vi "Test Queue Log Provider.vi"() -> (1 "pass?":bool)   [LabVIEW 2019, in "ANODE Tests.lvlib"]
uses:
  ANODE Tests.lvlib
  ANODE/Utility API/Queue Log Provider/impl/log_message.ctl
  ANODE/Utility API/Log Service/public/level.ctl
  34bea0a4-f80a-4efe-aaf4-9db1f3a8a041.vi
  4e885d52-342e-4d6f-86c2-bbc79adb3db9.vi
  901ffbec-7f76-4fda-a8b3-ab898965128c.vi
  31a8342b-9139-4bdf-bbc1-bb92f7179d80.vi
  c69379c1-06bc-43e8-abf1-6b6e803fbc34.vi
  7ff86ca6-88c0-4de2-a7d7-e18e6c48d840.vi
  f5e9308b-311a-4c07-9062-c62029aec88d.vi
  cd498dcc-2004-4e95-9cb1-3a88910e2f61.vi
  4bbd3971-874f-4069-8a4a-00f2533dc096.vi
  51edfdbb-9a3d-492a-8a02-2d0f54c6b824.vi
  8f198e5f-b4d0-4ca0-822a-d58fe651c8a2.vi
  ANODE/Util/Timestamp or now.vi
  ANODE/Utility API/Queue Log Provider/Queue Log Provider.lvclass
  ANODE/Utility API/Log Service/Log Service.lvclass
panel:
  out "expected output?":bool
  out "expected # of elements?":bool
  out "remaining elements":T1[](array[typedef]) {"level" items=["OFF"=0, "FATAL"=100, "ERROR"=200, "WARN"=300, "INFO"=400, "DEBUG"=500, "TRACE"=600, "ALL"=65535]}
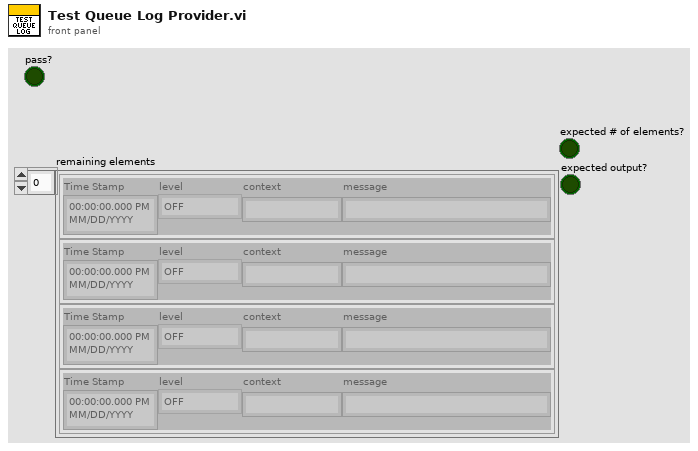
[diagram p1: front panel]
types:
  T1 = typedef "Utility API.lvlib/Queue Log Provider.lvclass/log_message.ctl" = cluster{"Time Stamp":timestamp, "level":T2, "context":string, "message":string}
  T2 = typedef "Utility API.lvlib/Log Service.lvclass/level.ctl" = u16
  T3 = typedef "LVCOOOP.lvlib/Support API.lvlib/Queue Log Provider.lvclass/log_message.ctl" = cluster{"Time Stamp":timestamp, "level":T4, "context":string, "message":string}
  T4 = typedef "LVCOOOP.lvlib/Support API.lvlib/Log Service.lvclass/level.ctl" = u16
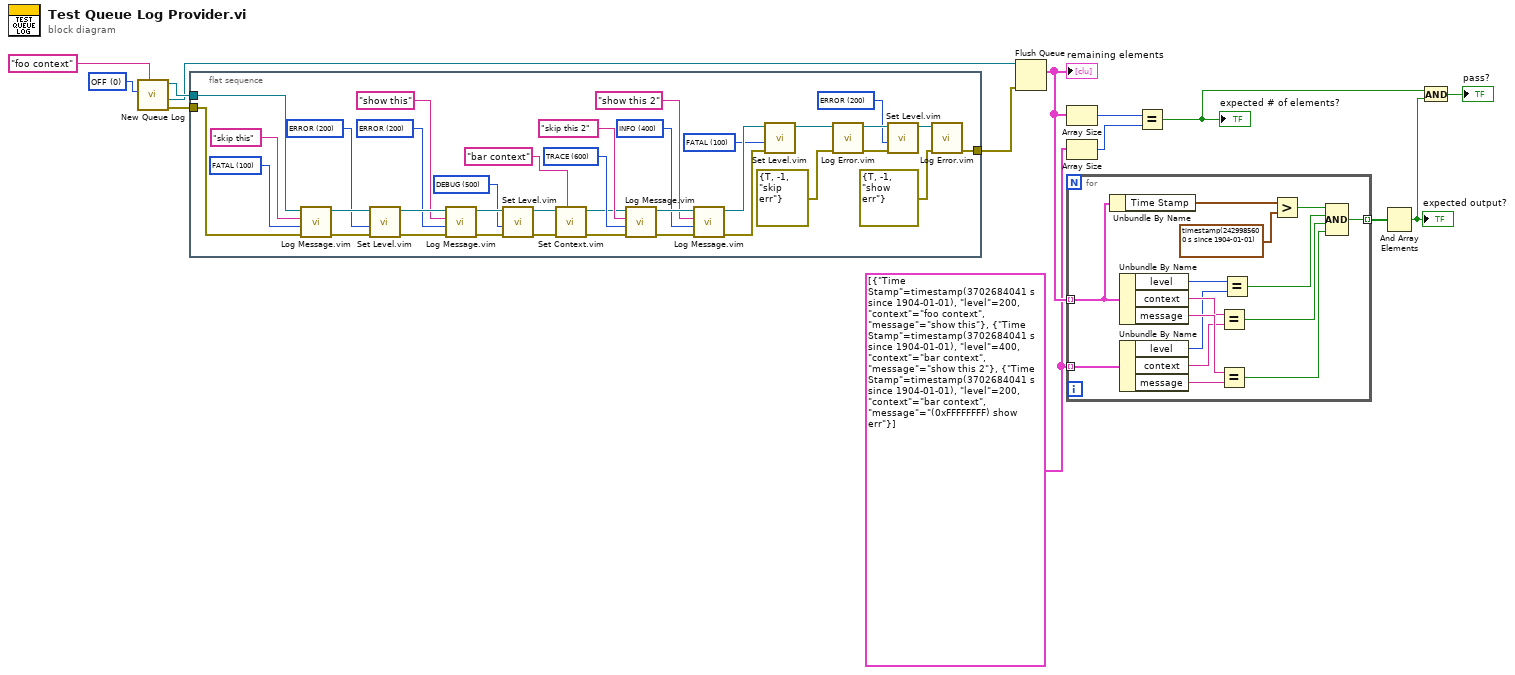
[diagram p0: block diagram]
diagram:
  w5 = T1[] [{"Time Stamp"=timestamp(3702684041.4619007 s since 1904-01-01), "level"=200, "context"="foo context", "message"="show this"}, {"Time Stamp"=timestamp(3702684041.4619007 s since 1904-01-01), "level"=400, "context"="bar context", "message"="show this 2"}, {"Time Stamp"=timestamp(3702684041.4619007 s since 1904-01-01), "level"=200, "context"="bar context", "message"="(0xFFFFFFFF) show err"}] ("remaining elements")
  w13 = T2 0 items=["OFF"=0, "FATAL"=100, "ERROR"=200, "WARN"=300, "INFO"=400, "DEBUG"=500, "TRACE"=600, "ALL"=65535] ("level")
  n1 = call "New Queue Log.vi"("context"="foo context", "level"=w13) -> ("error out"=w11:errorcluster, "queue out"=w9:refnum<queue>, "Queue Log Provider"=w12:refnum<data-value>)  [unwired: 7 in]
  n2 = flat-sequence {
    tunnel: w12 -> [w50]
    tunnel: w11 -> [w42]
    tunnel: [w19] -> w10
    frame #0 {
      w22 = T2 200 items=["OFF"=0, "FATAL"=100, "ERROR"=200, "WARN"=300, "INFO"=400, "DEBUG"=500, "TRACE"=600, "ALL"=65535] ("level")
      w27 = T2 100 items=["OFF"=0, "FATAL"=100, "ERROR"=200, "WARN"=300, "INFO"=400, "DEBUG"=500, "TRACE"=600, "ALL"=65535] ("level")
      w30 = T2 400 items=["OFF"=0, "FATAL"=100, "ERROR"=200, "WARN"=300, "INFO"=400, "DEBUG"=500, "TRACE"=600, "ALL"=65535] ("level")
      w34 = T2 600 items=["OFF"=0, "FATAL"=100, "ERROR"=200, "WARN"=300, "INFO"=400, "DEBUG"=500, "TRACE"=600, "ALL"=65535] ("level")
      w37 = T2 500 items=["OFF"=0, "FATAL"=100, "ERROR"=200, "WARN"=300, "INFO"=400, "DEBUG"=500, "TRACE"=600, "ALL"=65535] ("level")
      w43 = T2 200 items=["OFF"=0, "FATAL"=100, "ERROR"=200, "WARN"=300, "INFO"=400, "DEBUG"=500, "TRACE"=600, "ALL"=65535] ("level")
      w46 = T2 200 items=["OFF"=0, "FATAL"=100, "ERROR"=200, "WARN"=300, "INFO"=400, "DEBUG"=500, "TRACE"=600, "ALL"=65535] ("level")
      w49 = T2 100 items=["OFF"=0, "FATAL"=100, "ERROR"=200, "WARN"=300, "INFO"=400, "DEBUG"=500, "TRACE"=600, "ALL"=65535] ("level")
      n3 = call "Log Message.vim"("error in (no error)"=w42, "level"=w49, "message"="skip this", "Log Service in"=w50) -> ("error out"=w41:errorcluster, "Log Service out"=w47:refnum<data-value>)  [unwired: 6 in]
      n4 = call "Set Level.vim"("error in (no error)"=w41, "level"=w46, "Log Service in"=w47) -> ("error out"=w40:errorcluster, "Log Service out"=w45:refnum<data-value>)  [unwired: 7 in]
      n5 = call "Log Message.vim"("error in (no error)"=w40, "level"=w43, "message"="show this", "Log Service in"=w45) -> ("error out"=w38:errorcluster, "Log Service out"=w39:refnum<data-value>)  [unwired: 6 in]
      n6 = call "Set Level.vim"("error in (no error)"=w38, "level"=w37, "Log Service in"=w39) -> ("error out"=w17:errorcluster, "Log Service out"=w36:refnum<data-value>)  [unwired: 7 in]
      n7 = call "Set Context.vim"("context"="bar context", "error in (no error)"=w17, "Log Service in"=w36) -> ("error out"=w16:errorcluster, "Log Service out"=w18:refnum<data-value>)  [unwired: 7 in]
      n8 = call "Log Message.vim"("error in (no error)"=w16, "level"=w34, "message"="skip this 2", "Log Service in"=w18) -> ("error out"=w32:errorcluster, "Log Service out"=w33:refnum<data-value>)  [unwired: 6 in]
      n9 = call "Log Message.vim"("error in (no error)"=w32, "level"=w30, "message"="show this 2", "Log Service in"=w33) -> ("error out"=w29:errorcluster, "Log Service out"=w28:refnum<data-value>)  [unwired: 6 in]
      n10 = call "Set Level.vim"("error in (no error)"=w29, "level"=w27, "Log Service in"=w28) -> ("Log Service out"=w26:refnum<data-value>)  [unwired: 7 in, 1 out]
      n11 = call "Log Error.vim"("error in (no error)"=errorcluster {"status"=TRUE, "code"=-1, "source"="skip err"}, "Log Service in"=w26) -> ("error out"=w23:errorcluster, "Log Service out"=w24:refnum<data-value>)  [unwired: 8 in]
      n12 = call "Set Level.vim"("error in (no error)"=w23, "level"=w22, "Log Service in"=w24) -> ("Log Service out"=w21:refnum<data-value>)  [unwired: 7 in, 1 out]
      n13 = call "Log Error.vim"("error in (no error)"=errorcluster {"status"=TRUE, "code"=-1, "source"="show err"}, "Log Service in"=w21) -> ("error out"=w19:errorcluster)  [unwired: 8 in, 1 out]
    }
  }
  n14 = Flush Queue(queue=w9, error in (no error)=w10) -> (remaining elements=w6:T3[])  [unwired: 2 out]
  "remaining elements" <- w6
  n15 = Array Size(array=w6) -> (size(s)=w8:i32)
  n16 = Array Size(array=w5) -> (size(s)=w7:i32)
  n17 = for {
    tunnel: w6 -> [w63] mode=indexing
    tunnel: w5 -> [w62] mode=indexing
    tunnel: [w51] -> w4 mode=indexing
    n18 = Unbundle By Name(w63) -> ("Time Stamp"=w65:timestamp)
    n19 = Unbundle By Name(w63) -> ("level"=w57:T4, "context"=w58:string, "message"=w60:string)
    n20 = Unbundle By Name(w62) -> ("level"=w56:T2, "context"=w59:string, "message"=w61:string)
    n21 = Equal?(x=w58, y=w59) -> (x = y?=w53:bool)
    n22 = Equal?(x=w60, y=w61) -> (x = y?=w52:bool)
    n23 = Equal?(x=w57, y=w56) -> (x = y?=w54:bool)
    n24 = Greater?(x=w65, y=timestamp(2429985600 s since 1904-01-01)) -> (0:w55:bool)
    n25 = Compound Arithmetic op=AND(w55, w54, w53, w52) -> (w51:bool)
  }
  n26 = Equal?(x=w8, y=w7) -> (x = y?=w2:bool)
  "expected # of elements?" <- w2
  n27 = And Array Elements(Boolean array=w4) -> (logical AND=w3:bool)
  "expected output?" <- w3
  n28 = And(x=w2, y=w3) -> (x .and. y?=→"pass?":bool)
